vi "Helper - Number to Log String.vi"(9 "Input":dbl, 10 "Selector":string, 11 "PrevString":string) -> (3 "Output":string)   [LabVIEW 2011]
doc: "Part of Helper - Data to String.vi. Look there for more details."
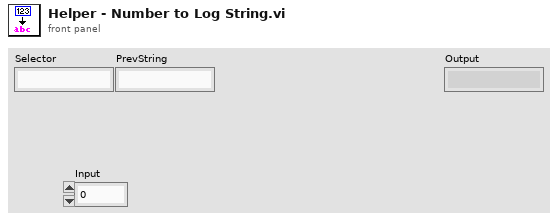
[diagram p1: front panel]
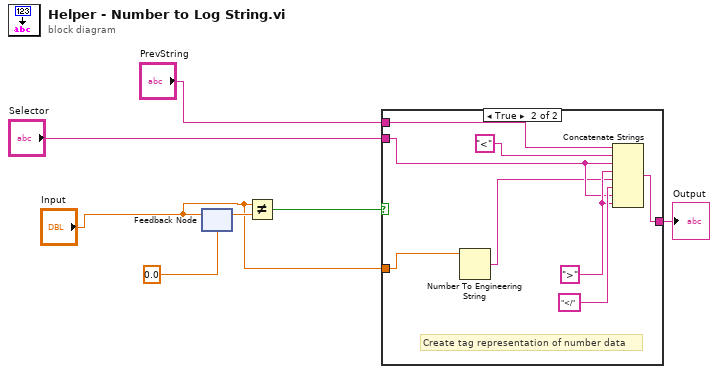
[diagram p0: block diagram]
diagram:
  n1 = feedback #1(0.0 ("Input")) -> (w5:dbl)
  n2 = feedback-in #1("Input") -> ()
  n3 = Not Equal?(x="Input", y=w5) -> (x != y?=w2:bool)
  n4 = case shown="True" w2 {
    tunnel: [w8 w16] -> w6
    tunnel: "Selector" -> [_ w11]
    tunnel: "Input" -> [_ w10]
    tunnel: "PrevString" -> [w8 w12]
    frame False {
    }
    frame True {
      w13 = ">" ("string")
      # "Create tag representation of number data"
      n5 = Number To Engineering String(4:w10) -> (0:w9:string)  [unwired: 3 in]
      n6 = Concatenate Strings(w12, "<" ("string"), w11, w13, w9, "</" ("string"), w11, w13) -> (w16:string)
    }
  }
  "Output" <- w6
